vi "gyroglobal.vi"(11 "Set(T)/Get(F)":bool=TRUE) -> (1 "Angular Rate":dbl, 3 "Angle":dbl)   [LabVIEW 2017]
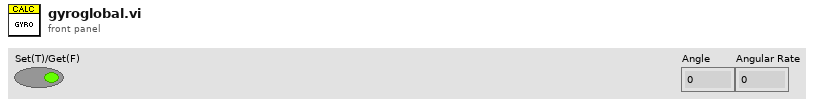
[diagram p1: front panel]
types:
  T1 = typedef "WPI_GyroDevRef.ctl" = cluster{"DevStatus":errorcluster, "Analog Channel":T2, "Gain (VoltsPerDegree/Second)":dbl, "Gyro Type":enum16{"Analog", "XRS450"}, "Handle":i32, "SPI Bus":T3, "Device Found":bool, "Sample Rate":dbl, "Calibrate On Open":bool, "Offset":dbl}
  T2 = typedef "FPGA_AIChannel.ctl" = enum8{"AI 0", "AI 1", "AI 2", "AI 3", "AI MXP 0", "AI MXP 1", "AI MXP 2", "AI MXP 3", "Invalid"}
  T3 = typedef "spi_bus.ctl" = enum16{"SPI On-Board, CS0", "SPI On-Board, CS1", "SPI On-Board, CS2", "SPI On-Board, CS3", "SPI MXP", "Invalid"}
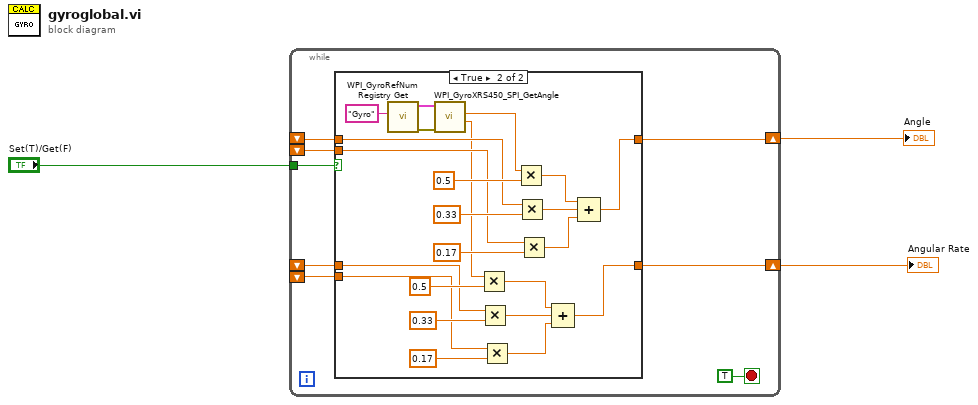
[diagram p0: block diagram]
diagram:
  n1 = while {
    shift-right: [w8] -> w2
    shift-left: _ -> [w10]
    shift-left: _ -> [w9]
    tunnel: "Set(T)/Get(F)" -> [w7]
    shift-right: [w6] -> w1
    shift-left: _ -> [w5]
    shift-left: _ -> [w4]
    stop <- TRUE stop-if-true
    n2 = case shown="True" w7 {
      tunnel: w10 -> [w13 w33]
      tunnel: w9 -> [_ w32]
      tunnel: [w13 w28] -> w8
      tunnel: [w12 w18] -> w6
      tunnel: w5 -> [w12 w16]
      tunnel: w4 -> [_ w15]
      frame False {
      }
      frame True {
        n3 = call <vilib>:"WPI_GyroRefNum Registry Get.vi"("refnum name"="Gyro") -> ("error out"=w27:errorcluster, "GyroDevRef"=w26:T1)  [unwired: 9 in]
        n4 = call <vilib>:"WPI_GyroXRS450_SPI_GetAngle.vi"("error in"=w27, "GyroDevRef"=w26) -> ("Angular Rate"=w17:dbl, "Angle"=w24:dbl)  [unwired: 5 in, 3 out]
        n5 = Multiply(x=w17, y=0.5) -> (x*y=w14:dbl)
        n6 = Multiply(x=w16, y=0.33) -> (x*y=w20:dbl)
        n7 = Multiply(x=w15, y=0.17) -> (x*y=w19:dbl)
        n8 = Multiply(x=w24, y=0.5) -> (x*y=w31:dbl)
        n9 = Multiply(x=w33, y=0.33) -> (x*y=w30:dbl)
        n10 = Multiply(x=w32, y=0.17) -> (x*y=w29:dbl)
        n11 = Compound Arithmetic op=ADD(w14, w20, w19) -> (w18:dbl)
        n12 = Compound Arithmetic op=ADD(w31, w30, w29) -> (w28:dbl)
      }
    }
  }
  "Angle" <- w2
  "Angular Rate" <- w1
